vi "vPage_9237x1_CHx4.vi"() -> ()   [LabVIEW 2022 SP3]
uses:
  <vilib>/Utility/sysdir.llb/System Directory Type.ctl
panel:
  in  "Show_FFT":bool
  out "C2":i32
  out "DAQ Stoped":bool
  out "C1":i32
  in  "SW \n(C1)":bool[](array[boolean])=[TRUE, FALSE, FALSE, FALSE, TRUE, TRUE, TRUE, TRUE]
  in  "Sample \nto Read":i32=2000
  in  "Sample\nRate":dbl=2000.0
  in  "¸ê®Æ§¨\nµù°O>":string
  in  "Enable Saving":bool
  in  "Stop":bool
  out "C1-Save":bool
  out "C1-Trigger":bool
  out "C1-All":dynamicdata(graph)
  out "C1-0":dynamicdata(graph)
  out "C1-2":dynamicdata(graph)
  out "C1-1":dynamicdata(graph)
  out "C1-3":dynamicdata(graph)
  # "使用前請先確認 \nDAQ 擷取卡設定"
  # "本頁畫面顯示為 觸發後訊號"
  # "FFT Filter by useing High-pass with Lower Cut-Off (Hz)"
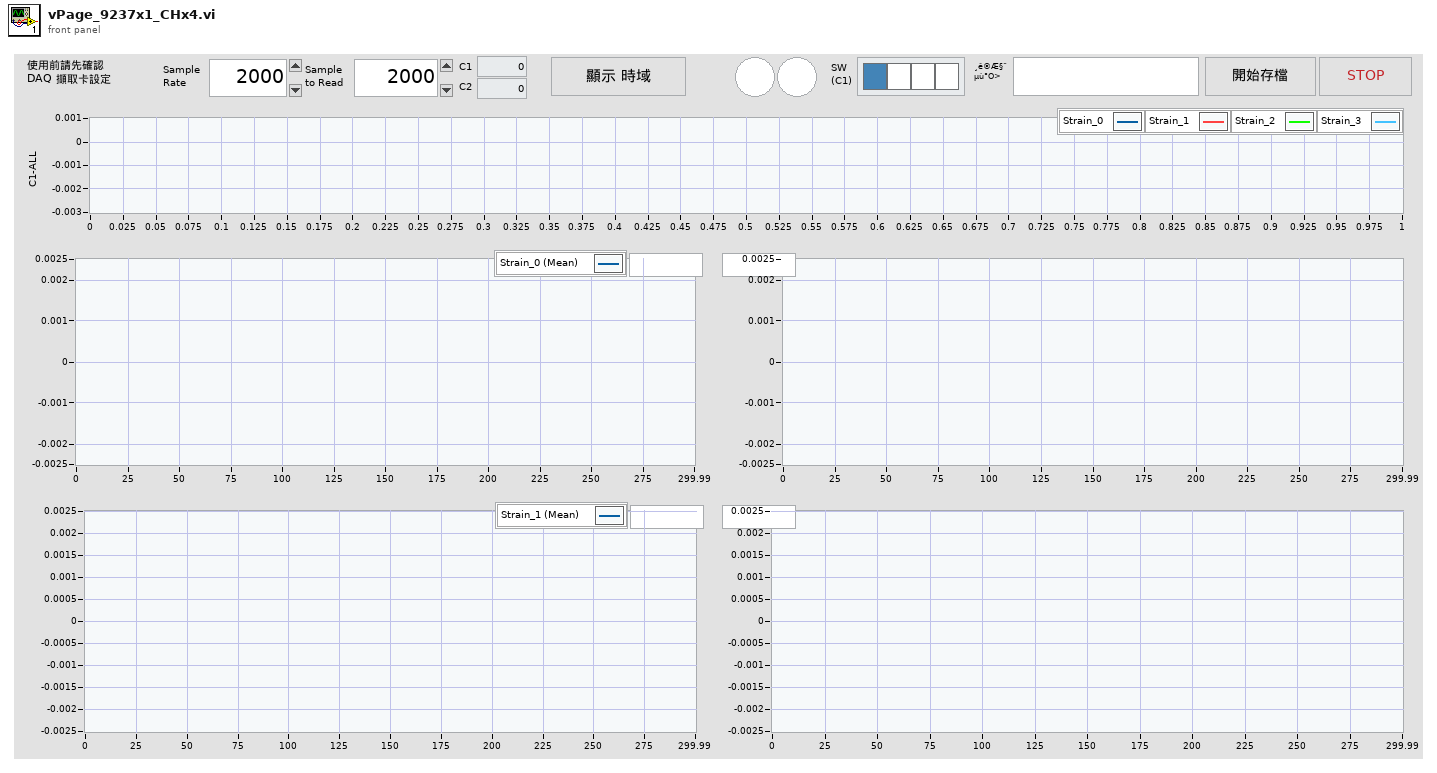
[diagram p1: front panel]
types:
  T1 = enum8{"Enabled", "Disabled", "Disabled and Grayed Out"}
  T2 = typedef "System Directory Type.ctl" = i32
  T3 = cluster{"task out":refnum<k21>, "data":dynamicdata}
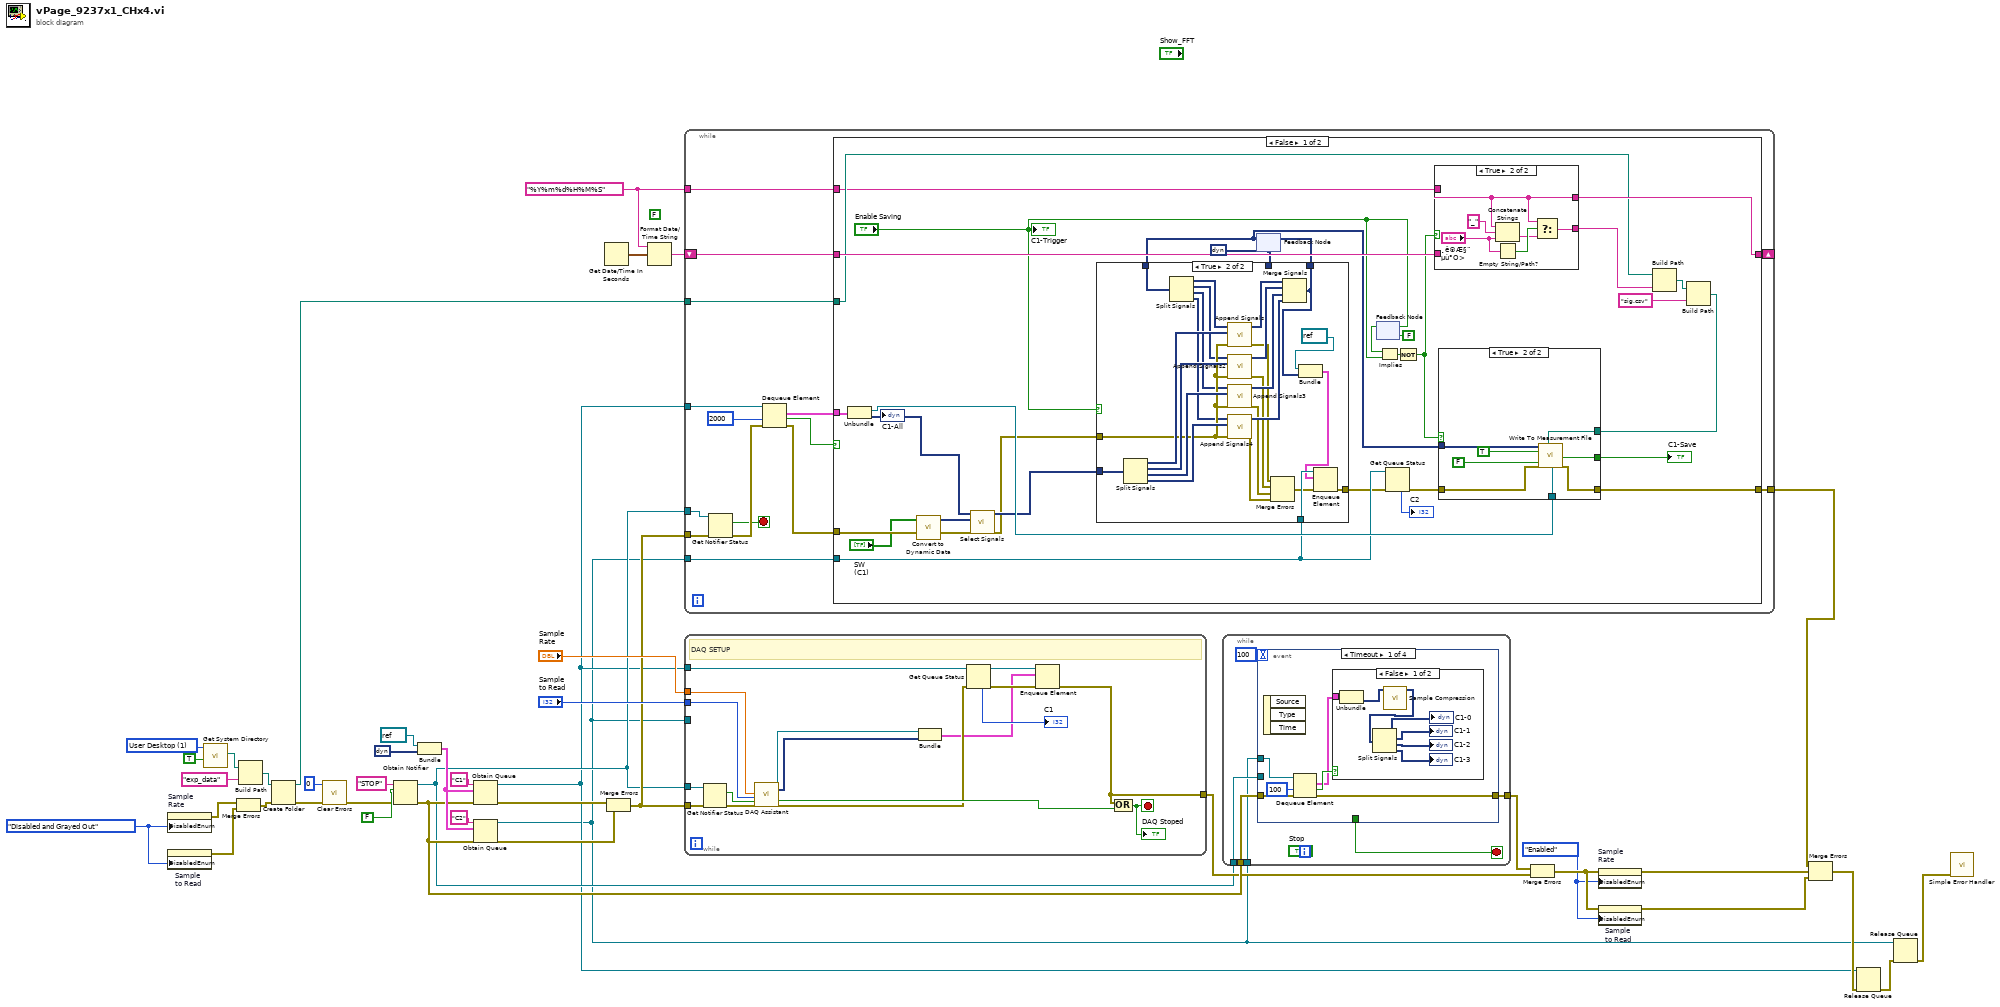
[diagram p0: block diagram]
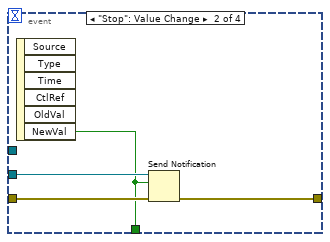
[diagram p3: hidden frame]
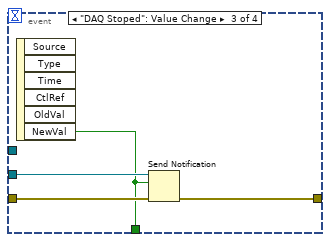
[diagram p4: hidden frame]
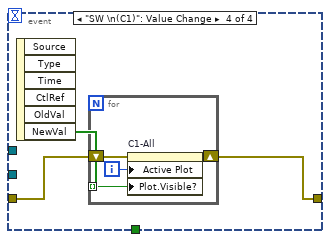
[diagram p5: hidden frame]
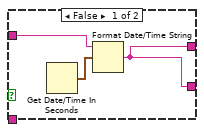
[diagram p8: hidden frame]
diagram:
  (unwired) FALSE
  w9 = T1."Enabled" ("Disabled")
  w14 = T1."Disabled and Grayed Out" ("Disabled")
  w15 = "%Y%m%d%H%M%S" ("time format string (%c)")
  w25 = T2 1 items=["User Home"=0, "User Desktop"=1, "User Documents"=2, "User Application Data"=3, "User Preferences"=4, "User Temporary"=5, "Public Documents"=6, "Public Application Data"=7, "Public Preferences"=8, "Public Cache"=13, "System Core Libraries"=9, "System Installed Libraries"=10, "Application Files"=11, "Boot Volume Root"=12] ("system directory type")
  n1 = property on="Sample\nRate" class="DigNum (strict)"("DisabledEnum"=w14) -> (error out=w13:errorcluster)  [unwired: 2 in, 1 out]
  n2 = property on="Sample \nto Read" class="DigNum (strict)"("DisabledEnum"=w14) -> (error out=w11:errorcluster)  [unwired: 2 in, 1 out]
  n3 = call <vilib>:"Get System Directory.vi"("create directory if not found? (F)"=TRUE, "system directory type"=w25) -> ("system directory"=w27:path)  [unwired: 9 in]
  n4 = Merge Errors(w13, w11) -> (w12:errorcluster)
  n5 = Build Path(base path=w27, name or relative path="exp_data") -> (appended path=w21:path)
  n6 = Create Folder(path (use dialog)=w21, error in=w12) -> (created path=w20:path, error out=w23:errorcluster)  [unwired: 1 in, 1 out]
  n7 = call <vilib>:"Clear Errors.vi"("error in (no error)"=w23, "specific error code to clear (0: all)"=0) -> ("error out"=w22:errorcluster)  [unwired: 4 in, 1 out]
  n8 = Obtain Notifier(name (unnamed)="STOP", notification data type=FALSE, error in (no error)=w22) -> (notifier out=w16:refnum<notifier>, error out=w19:errorcluster)  [unwired: 1 in, 1 out]
  n9 = Bundle("task out"=refnum<k21> refnum, "data"=dynamicdata []) -> (w32:T3)  [unwired: 1 in]
  n10 = Obtain Queue(name (unnamed)="C1", element data type=w32, error in (no error)=w19) -> (queue out=w2:refnum<queue>, error out=w42:errorcluster)  [unwired: 2 in, 1 out]
  n11 = Obtain Queue(name (unnamed)="C2", element data type=w32, error in (no error)=w19) -> (queue out=w1:refnum<queue>, error out=w41:errorcluster)  [unwired: 2 in, 1 out]
  n12 = Get Date/Time In Seconds() -> (seconds since 1Jan1904=w30:timestamp)
  n13 = Merge Errors(w42, w41) -> (w31:errorcluster)
  n14 = Format Date/Time String(time format string (%c)=w15, seconds (now)=w30) -> (date/time string=w29:string)  [unwired: 1 in]
  n15 = while {
    tunnel: w31 -> [w57]
    tunnel: w16 -> [w55]
    tunnel: w2 -> [w54]
    tunnel: w1 -> [w43]
    shift-right: [w48] -> _
    shift-left: w29 -> [w49]
    tunnel: w20 -> [w47]
    tunnel: [w46] -> w3
    tunnel: w15 -> [w44]
    stop <- w45 stop-if-true
    n16 = Get Notifier Status(notifier=w55, error in (no error)=w57) -> (current notification=w45:bool, error out=w56:errorcluster)  [unwired: 3 out]
    n17 = Dequeue Element(queue=w54, timeout in ms (-1)=2000, error in (no error)=w56) -> (element=w51:T3, timed out?=w52:bool, error out=w50:errorcluster)  [unwired: 1 out]
    n18 = case shown="False" w52 {
      tunnel: w51 -> [w87 _]
      tunnel: w50 -> [w86 w133]
      tunnel: w49 -> [w82 w134]
      tunnel: [w81 w134] -> w48
      tunnel: w47 -> [w80 _]
      tunnel: [w62 w133] -> w46
      tunnel: w44 -> [w72 _]
      tunnel: w43 -> [w61 _]
      frame False {
        w71 = dynamicdata [] ("Waveform Graph")
        n19 = Unbundle(w87) -> ("task out"=w84:refnum<k21>, "data"=w85:dynamicdata)
        "C1-All" <- w85
        n20 = call "Convert to Dynamic Data"("Array"="SW \n(C1)") -> ("Dynamic Data Type"=w74:dynamicdata)  [unwired: 3 in]
        n21 = call "Select Signals"("error in (no error)"=w86, "Selector Input"=w74, "Signals"=w85) -> ("error out"=w69:errorcluster, "Signal Out"=w83:dynamicdata)  [unwired: 7 in]
        n22 = feedback #1(w71) -> (w63:dynamicdata)
        n23 = case shown="True" "Enable Saving" {
          tunnel: w83 -> [_ w123]
          tunnel: w69 -> [w97 w118]
          tunnel: w63 -> [_ w105]
          tunnel: [w98 w103] -> w64
          tunnel: w71 -> [w98 _]
          tunnel: [w97 w99] -> w60
          tunnel: w61 -> [_ w102]
          frame False {
          }
          frame True {
            n24 = Split Signals(w123) -> (w119:dynamicdata, w120:dynamicdata, w121:dynamicdata, w122:dynamicdata)  [unwired: 4 in]
            n25 = Split Signals(w105) -> (w110:dynamicdata, w111:dynamicdata, w112:dynamicdata, w113:dynamicdata)  [unwired: 4 in]
            n26 = call "Append Signals"("error in (no error)"=w118, "Input Signal B"=w119, "Input Signal A"=w110) -> ("error out"=w109:errorcluster, "Appended Signals"=w117:dynamicdata)  [unwired: 7 in]
            n27 = call "Append Signals2"("error in (no error)"=w118, "Input Signal B"=w120, "Input Signal A"=w111) -> ("error out"=w108:errorcluster, "Appended Signals"=w116:dynamicdata)  [unwired: 7 in]
            n28 = call "Append Signals3"("error in (no error)"=w118, "Input Signal B"=w121, "Input Signal A"=w112) -> ("error out"=w107:errorcluster, "Appended Signals"=w115:dynamicdata)  [unwired: 7 in]
            n29 = call "Append Signals4"("error in (no error)"=w118, "Input Signal B"=w122, "Input Signal A"=w113) -> ("error out"=w106:errorcluster, "Appended Signals"=w114:dynamicdata)  [unwired: 7 in]
            n30 = Merge Errors(w109, w108, w107, w106) -> (w101:errorcluster)
            n31 = Merge Signals(w117, w116, w115, w114) -> (w103:dynamicdata)
            n32 = Bundle("task out"=refnum<k21> refnum, w103) -> (w100:cluster{"task out":refnum<k21>, dynamicdata})  [unwired: 1 in]
            n33 = Enqueue Element(queue=w102, element=w100, error in (no error)=w101) -> (error out=w99:errorcluster)  [unwired: 1 in, 2 out]
          }
        }
        n34 = feedback-in #1(w64) -> ()
        n35 = feedback-in #2("Enable Saving") -> ()
        n36 = feedback #2(FALSE ("Enable Saving")) -> (w68:bool)
        n37 = Implies(1:"Enable Saving", 2:w68) -> (0:w70:bool)
        n38 = Get Queue Status(queue=w61, error in (no error)=w60) -> (error out=w59:errorcluster, # elements in queue=→"C2":i32)  [unwired: 1 in, 6 out]
        n39 = Not(x=w70) -> (.not. x?=w65:bool)
        n40 = case shown="True" w65 {
          tunnel: [w124 w127] -> w81
          tunnel: w82 -> [_ w127]
          tunnel: [w124 w129] -> w73
          tunnel: w72 -> [w125 _]
          frame False {
            n41 = Get Date/Time In Seconds() -> (seconds since 1Jan1904=w126:timestamp)
            n42 = Format Date/Time String(time format string (%c)=w125, seconds (now)=w126) -> (date/time string=w124:string)  [unwired: 1 in]
          }
          frame True {
            n43 = Concatenate Strings(w127, "_" ("string"), "¸ê®Æ§¨\nµù°O>") -> (w130:string)
            n44 = Empty String/Path?(string/path="¸ê®Æ§¨\nµù°O>") -> (empty?=w131:bool)
            n45 = Select(t=w127, s=w131, f=w130) -> (s? t:f=w129:string)
          }
        }
        n46 = Build Path(base path=w80, name or relative path=w73) -> (appended path=w79:path)
        n47 = Build Path(base path=w79, name or relative path="sig.csv") -> (appended path=w77:path)
        n48 = case shown="True" w65 {
          tunnel: w84 -> [_ w96]
          tunnel: w77 -> [_ w95]
          tunnel: [_ w94] -> w76
          tunnel: w63 -> [_ w92]
          tunnel: w59 -> [w88 w90]
          tunnel: [w88 w89] -> w62
          frame False {
          }
          frame True {
            n49 = call "Write To Measurement File"("Signals"=w92, "Enable"=TRUE, "new_file"=FALSE, "error in (no error)"=w90, "Filename"=w95, "DAQmx Task"=w96) -> ("Saving Data"=w94:bool, "error out"=w89:errorcluster)  [unwired: 11 in, 1 out]
          }
        }
        "C1-Save" <- w76
        "C1-Trigger" <- "Enable Saving"
      }
      frame True {
      }
    }
  }
  n50 = while {
    tunnel: [w146] -> w17
    tunnel: w1 -> [_]
    tunnel: w2 -> [w143]
    tunnel: w31 -> [w142]
    tunnel: w16 -> [w141]
    tunnel: "Sample \nto Read" -> [w137]
    tunnel: "Sample\nRate" -> [w136]
    stop <- w144 stop-if-true
    # "DAQ SETUP"
    n51 = Get Notifier Status(notifier=w141, error in (no error)=w142) -> (current notification=w150:bool, error out=w151:errorcluster)  [unwired: 3 out]
    n52 = call "DAQ Assistant"("rate"=w136, "number of samples"=w137, "error in"=w151, "stop (F)"=w150) -> ("task out"=w139:refnum<k21>, "data"=w135:dynamicdata, "stopped"=w149:bool, "error out"=w147:errorcluster)  [unwired: 12 in]
    n53 = Bundle("task out"=w139, "data"=w135) -> (w138:T3)  [unwired: 1 in]
    n54 = Get Queue Status(queue=w143, error in (no error)=w147) -> (queue out=w140:refnum<queue>, error out=w148:errorcluster, # elements in queue=→"C1":i32)  [unwired: 1 in, 5 out]
    n55 = Enqueue Element(queue=w140, element=w138, error in (no error)=w148) -> (error out=w146:errorcluster)  [unwired: 1 in, 2 out]
    n56 = Compound Arithmetic op=OR(w146, w149) -> (w144:bool)
    "DAQ Stoped" <- w144
  }
  n57 = while {
    tunnel: w19 -> [w157]
    tunnel: [w156] -> w18
    tunnel: w16 -> [w155]
    tunnel: w1 -> [w152]
    stop <- w154 stop-if-true
    n58 = event shown="[0] Timeout" {
      selector: _ -> [_ _ _ _]
      dyn-events: _ -> [_ _ _ _]
      timeout: 100 -> [_ _ _ _]
      tunnel: w157 -> [w162 w174 w178 w181]
      tunnel: [w161 w173 w177 w180] -> w156
      tunnel: w155 -> [_ w172 w176 _]
      tunnel: [_ w171 w175 _] -> w154
      tunnel: w152 -> [w163 _ _ _]
      event Timeout {
        n59 = event-data() -> ()  [unwired: 1 in, 3 out]
        n60 = Dequeue Element(queue=w163, timeout in ms (-1)=100, error in (no error)=w162) -> (element=w158:T3, timed out?=w159:bool, error out=w161:errorcluster)  [unwired: 1 out]
        n61 = case shown="False" w159 {
          tunnel: w158 -> [w170 _]
          frame False {
            n62 = Unbundle(w170) -> ("data"=w165:dynamicdata)  [unwired: 1 out]
            n63 = call "Sample Compression"("Signals"=w165) -> ("Mean"=w164:dynamicdata)  [unwired: 8 in, 2 out]
            n64 = Split Signals(w164) -> (→"C1-0":dynamicdata, →"C1-1":dynamicdata, →"C1-2":dynamicdata, →"C1-3":dynamicdata)  [unwired: 4 in]
          }
          frame True {
          }
        }
      }
      event "Stop": Value Change {
        n65 = event-data() -> ("NewVal"=w171:bool)  [unwired: 1 in, 5 out]
        n66 = Send Notification(notification=w171, notifier=w172, error in (no error)=w174) -> (error out=w173:errorcluster)  [unwired: 1 out]
      }
      event "DAQ Stoped": Value Change {
        n67 = event-data() -> ("NewVal"=w175:bool)  [unwired: 1 in, 5 out]
        n68 = Send Notification(notification=w175, notifier=w176, error in (no error)=w178) -> (error out=w177:errorcluster)  [unwired: 1 out]
      }
      event "SW \n(C1)": Value Change {
        n69 = event-data() -> ("NewVal"=w179:bool[])  [unwired: 1 in, 5 out]
        n70 = for {
          shift-right: [w184] -> w180
          shift-left: w181 -> [w185]
          tunnel: w179 -> [w182] mode=indexing
          i -> [w183]
          n71 = property on="C1-All" class="WFGraph (strict)"(error in=w185, "Active Plot"=w183, "Plot.Visible?"=w182) -> (error out=w184:errorcluster)  [unwired: 1 in, 1 out]
        }
      }
    }
  }
  n72 = Merge Errors(w18, w17) -> (w10:errorcluster)
  n73 = property on="Sample\nRate" class="DigNum (strict)"(error in=w10, "DisabledEnum"=w9) -> (error out=w8:errorcluster)  [unwired: 1 in, 1 out]
  n74 = property on="Sample \nto Read" class="DigNum (strict)"(error in=w10, "DisabledEnum"=w9) -> (error out=w7:errorcluster)  [unwired: 1 in, 1 out]
  n75 = Merge Errors(w3, w8, w7) -> (w4:errorcluster)
  n76 = Release Queue(queue=w2, error in (no error)=w4) -> (error out=w5:errorcluster)  [unwired: 1 in, 2 out]
  n77 = Release Queue(queue=w1, error in (no error)=w5) -> (error out=w6:errorcluster)  [unwired: 1 in, 2 out]
  n78 = call <vilib>:"Simple Error Handler.vi"("error in (no error)"=w6) -> ()  [unwired: 4 in, 5 out]
